vi "variable_W.vi"(4 "永久生成在本地（F）":bool, 6 "附加的Information":T1={"YT_TYPE"=enum."Array_COMBO", "TypeData"=[], "Tips"=""}, 8 "error in (no error)":errorcluster, 9 "待写入池的输入控件":variant, 10 "待写入池变量名称":string, 11 "函数池名称 in":i32) -> (0 "error out":errorcluster, 2 "待写入池变量名称out":string, 3 "函数池名称 out":i32)   [LabVIEW 2017]
doc: "YYLL VarSystem"
uses:
  variable_W.ctl
  YtCommon.lvlibp/yt`Data-Ytester Type Data.ctl
  YtCommon.lvlibp
panel:
  # "非重入避免写本地竞争！"
  # "TypeData约定：\n枚举、Radio Buttons填items[]\ncmbbox填items[]后加文本1或0\n表示允许未定义详见图片"
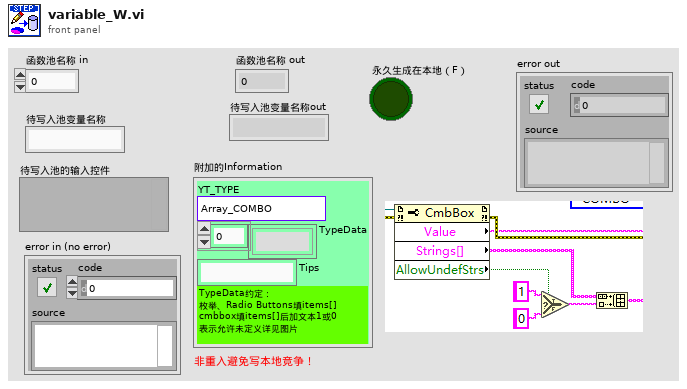
[diagram p1: front panel]
types:
  T1 = typedef "variable_W.ctl" = cluster{"YT_TYPE":T2, "TypeData":string[], "Tips":string}
  T2 = typedef "YtCommon.lvlibp/yt`Data-Ytester Type Data.ctl" = enum16{"NULL", "NUM", "BOOL", "TXT", "ENUM", "TIME", "PATH", "VISA", "COMBO", "ColorBox", "RadioBtn", "Array_NUM", "Array_BOOL", "Array_TXT", "Array_ENUM", "Array_PATH", "Array_COMBO"}
  T3 = cluster{"YT_TYPE":T2, "TypeData":string, "Tips":string}
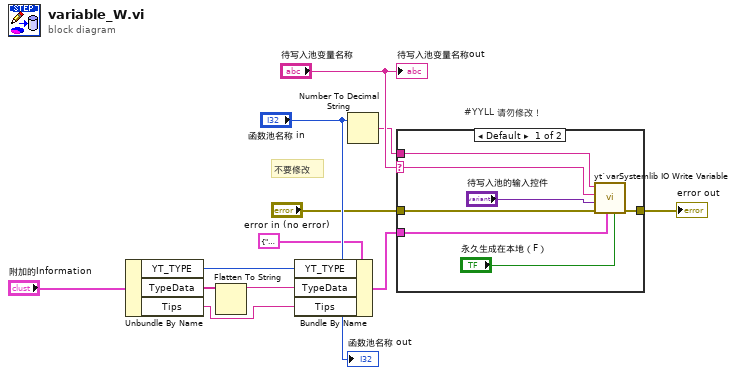
[diagram p0: block diagram]
diagram:
  # "不要修改"
  # "#YYLL 请勿修改！"
  n1 = Unbundle By Name("附加的Information") -> ("YT_TYPE"=w4:T2, "TypeData"=w3:string[], "Tips"=w1:string)
  n2 = Flatten To String(anything=w3) -> (data string=w2:string)  [unwired: 3 in, 2 out]
  n3 = Bundle By Name(cluster=T3 {"YT_TYPE"=enum."NULL", "TypeData"="", "Tips"=""} ("附加的Information 对内"), "YT_TYPE"=w4, "TypeData"=w2, "Tips"=w1) -> (w6:T3)
  n4 = Number To Decimal String(number="函数池名称 in") -> (decimal integer string=w9:string)  [unwired: 1 in]
  n5 = case shown="Default" "待写入池变量名称" {
    selector: "待写入池变量名称" -> [w15 _]
    tunnel: [w17 w20] -> w8
    tunnel: "error in (no error)" -> [w18 w20]
    tunnel: w6 -> [w14 _]
    tunnel: w9 -> [w16 _]
    frame Default {
      n6 = call "yt`varSystemlib IO Write Variable.vi"("永久生成在本地（F）"="永久生成在本地（F）", "附加的Information"=w14, "error in (no error)"=w18, "待写入数据"="待写入池的输入控件", "变量名称"=w15, "池名称"=w16) -> ("error out"=w17:errorcluster)  [unwired: 3 in, 2 out]
    }
    frame "" {
    }
  }
  "error out" <- w8
  "函数池名称 out" <- "函数池名称 in"
  "待写入池变量名称out" <- "待写入池变量名称"
